vi "linear_ramp_with_sinusoidal_return_and_phase_shift_multiD.vi"(0 "Left Padding":u32, 1 "Sweep Time (µs)":u32, 2 "Amplitude":dbl, 3 "Offset":dbl, 4 "Sweep Interval (µS)":u32, 5 "Number of Slices":u32, 6 "Right Padding":u32) -> (16 "output array":dbl[](array[numeric]))   [LabVIEW 2012]
uses:
  <vilib>/Analysis/1siggen.llb/Ramp Pattern by Samples.vi
  <vilib>/Analysis/NI_AALBase.lvlib
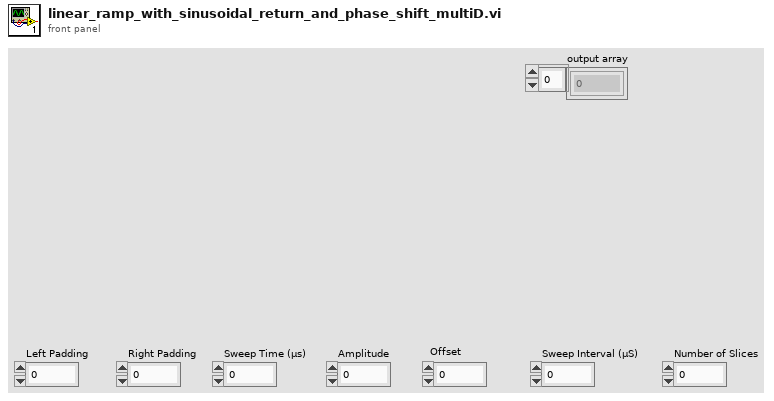
[diagram p1: front panel]
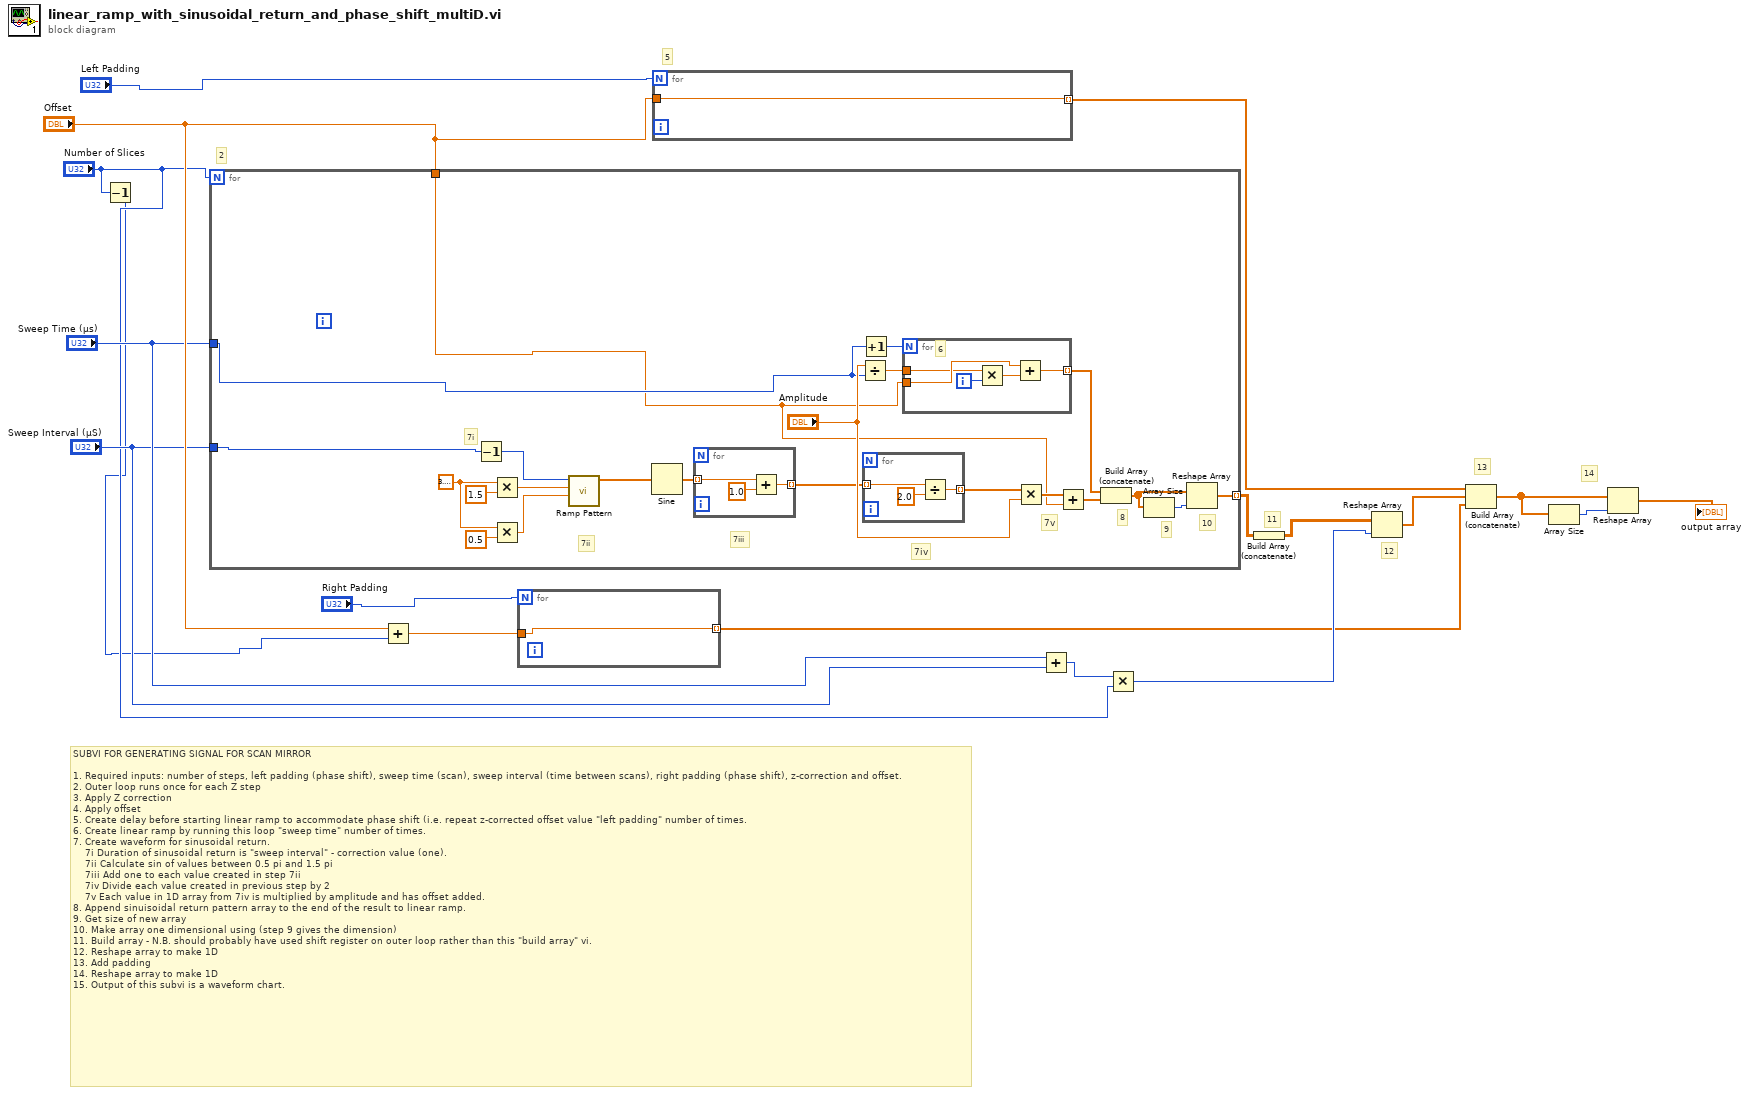
[diagram p0: block diagram]
diagram:
  # "14"
  # "13"
  # "12"
  # "11"
  # "5"
  # "2"
  # "SUBVI FOR GENERATING SIGNAL FOR SCAN MIRROR\n\n1. Required inputs: number of steps, left padding (phase shift), sweep time (scan), sweep interval (time between scans), right padding (phase shift), z-correction and offset.\n2. Outer loop runs once for each Z step\n3. Apply Z correction\n4. Apply offset\n5. Create delay before starting linear ramp to accommodate phase shift (i.e. repeat z-corrected offset value \"left padding\" number of times.\n6. Create linear ramp by running this loop \"sweep time\" number of times.\n7. Create waveform for sinusoidal return.\n    7i Duration of sinusoidal return is \"sweep interval\" - correction value (one). \n    7ii Calculate sin of values between 0.5 pi and 1.5 pi\n    7iii Add one to each value created in step 7ii\n    7iv Divide each value created in previous step by 2\n    7v Each value in 1D array from 7iv is multiplied by amplitude and has offset added.\n8. Append sinuisoidal return pattern array to the end of the result to linear ramp.\n9. Get size of new array\n10. Make array one dimensional using (step 9 gives the dimension)\n11. Build array - N.B. should probably have used shift register on outer loop rather than this \"build array\" vi.\n12. Reshape array to make 1D\n13. Add padding\n14. Reshape array to make 1D\n15. Output of this subvi is a waveform chart."
  n1 = Decrement(x="Number of Slices") -> (x-1=w1:u32)
  n2 = for {
    N: "Number of Slices" -> [_]
    tunnel: "Sweep Interval (µS)" -> [w20]
    tunnel: "Sweep Time (µs)" -> [w21]
    tunnel: "Offset" -> [w19]
    tunnel: [w22] -> w14 mode=indexing
    w36 = 3.141592653589793
    # "10"
    # "9"
    # "8"
    # "7v"
    # "7iv"
    # "7iii"
    # "7ii"
    # "7i"
    n3 = Decrement(x=w20) -> (x-1=w26:u32)
    n4 = Multiply(x=w36, y=1.5) -> (x*y=w32:dbl)
    n5 = Multiply(x=w36, y=0.5) -> (x*y=w33:dbl)
    n6 = call-poly <vilib>:"Ramp Pattern.vi"("start"=w33, "end"=w32, "samples"=w26) -> ("Ramp Pattern"=w31:dbl[])  [unwired: 7 in, 1 out]
    n7 = Sine(x=w31) -> (sin(x)=w29:dbl[])
    n8 = for {
      tunnel: w29 -> [w46] mode=indexing
      tunnel: [w45] -> w28 mode=indexing
      n9 = Add(x=w46, y=1.0) -> (x+y=w45:dbl)
    }
    n10 = Divide(x="Amplitude", y=w21) -> (x/y=w39:dbl)
    n11 = Increment(x=w21) -> (x+1=w37:u32)
    n12 = for {
      tunnel: w28 -> [w43] mode=indexing
      tunnel: [w42] -> w27 mode=indexing
      n13 = Divide(x=w43, y=2.0) -> (x/y=w42:dbl)
    }
    n14 = for {
      N: w37 -> [_]
      tunnel: w19 -> [w51]
      tunnel: w39 -> [w49]
      tunnel: [w47] -> w38 mode=indexing
      i -> [w50]
      # "6"
      n15 = Multiply(x=w49, y=w50) -> (x*y=w48:dbl)
      n16 = Add(x=w51, y=w48) -> (x+y=w47:dbl)
    }
    n17 = Multiply(x=w27, y="Amplitude") -> (x*y=w30:dbl[])
    n18 = Add(x=w30, y=w19) -> (x+y=w25:dbl[])
    n19 = Build Array (concatenate)(w38, w25) -> (w24:dbl[])
    n20 = Array Size(array=w24) -> (size(s)=w23:i32)
    n21 = Reshape Array(w24, w23) -> (w22:dbl[])
  }
  n22 = Add(x="Offset", y=w1) -> (x+y=w15:dbl)
  n23 = for {
    N: "Right Padding" -> [_]
    tunnel: w15 -> [w52]
    tunnel: [w52] -> w6 mode=indexing
  }
  n24 = for {
    N: "Left Padding" -> [_]
    tunnel: "Offset" -> [w53]
    tunnel: [w53] -> w8 mode=indexing
  }
  n25 = Add(x="Sweep Time (µs)", y="Sweep Interval (µS)") -> (x+y=w10:u32)
  n26 = Multiply(x=w10, y="Number of Slices") -> (x*y=w9:u32)
  n27 = Build Array (concatenate)(w14) -> (w13:dbl[][])
  n28 = Reshape Array(w13, w9) -> (w7:dbl[])
  n29 = Build Array (concatenate)(w8, w7, w6) -> (w5:dbl[])
  n30 = Array Size(array=w5) -> (size(s)=w4:i32)
  n31 = Reshape Array(w5, w4) -> (→"output array":dbl[])
